vi "Execute.vi"(8 "error in (no error)":errorcluster, 10 "Plugin Display UI in":refnum<class "Plugin Display UI.lvclass">, 11 "Plugin Handler Shifter Data Definition":T1) -> (0 "error out":errorcluster, 1 "Stop?":bool, 2 "Plugin Generic Command out":refnum<class "Plugin Handler Command.lvclass">, 3 "Plugin Handler Shifter Data Out":T1)   [LabVIEW 2011, in "Plugin Display UI.lvclass"]
uses:
  Plugin Display UI.lvclass
  Plugin Handler Command.lvclass
  Plugin Strict Type Definitions/Plugin Handler Shifter Data Definition.ctl
  Parent Plugin Definition/Plugin Template/Generic Plugin.lvclass
  Plugin Strict Type Definitions/Plugin Configuration Information.ctl
  User Interface/UI Command Manager/UI Command Manager.lvclass
  User Interface/UI Command Manager/UI Set Header Text/Set Header Text.lvclass
  User Interface/UI Command Manager/UI Load SubPanel Display/UI Load SubPanel Display.lvclass
  User Interface/UI Command Manager/UI Slide Panel/Slide Panel Off Screen.lvclass
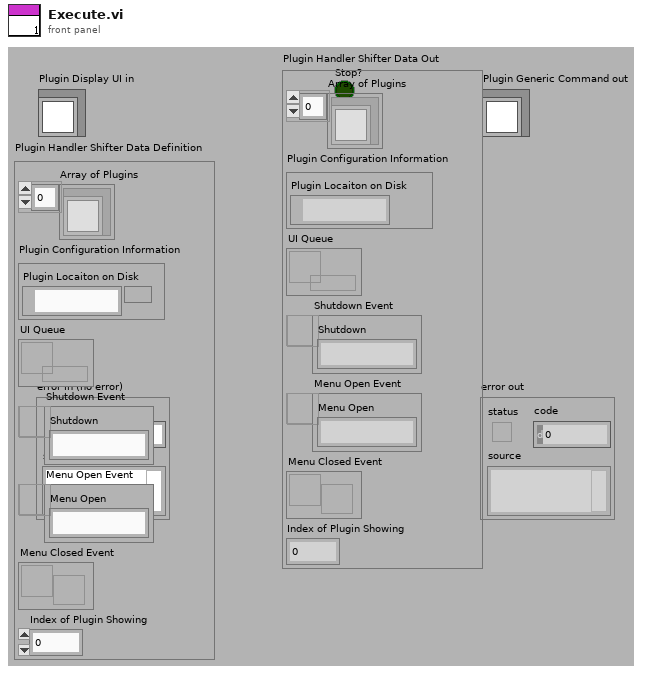
[diagram p1: front panel]
types:
  T1 = typedef "Plugin Handler Shifter Data Definition.ctl" = cluster{"Array of Plugins":refnum<class "Generic Plugin.lvclass">[], "Plugin Configuration Information":T2, "UI Queue":refnum<queue>, "Shutdown Event":refnum<user-event>, "Menu Open Event":refnum<user-event>, "Menu Closed Event":refnum<user-event>, "Index of Plugin Showing":i32}
  T2 = typedef "Plugin Configuration Information.ctl" = cluster{"Plugin Locaiton on Disk":path}
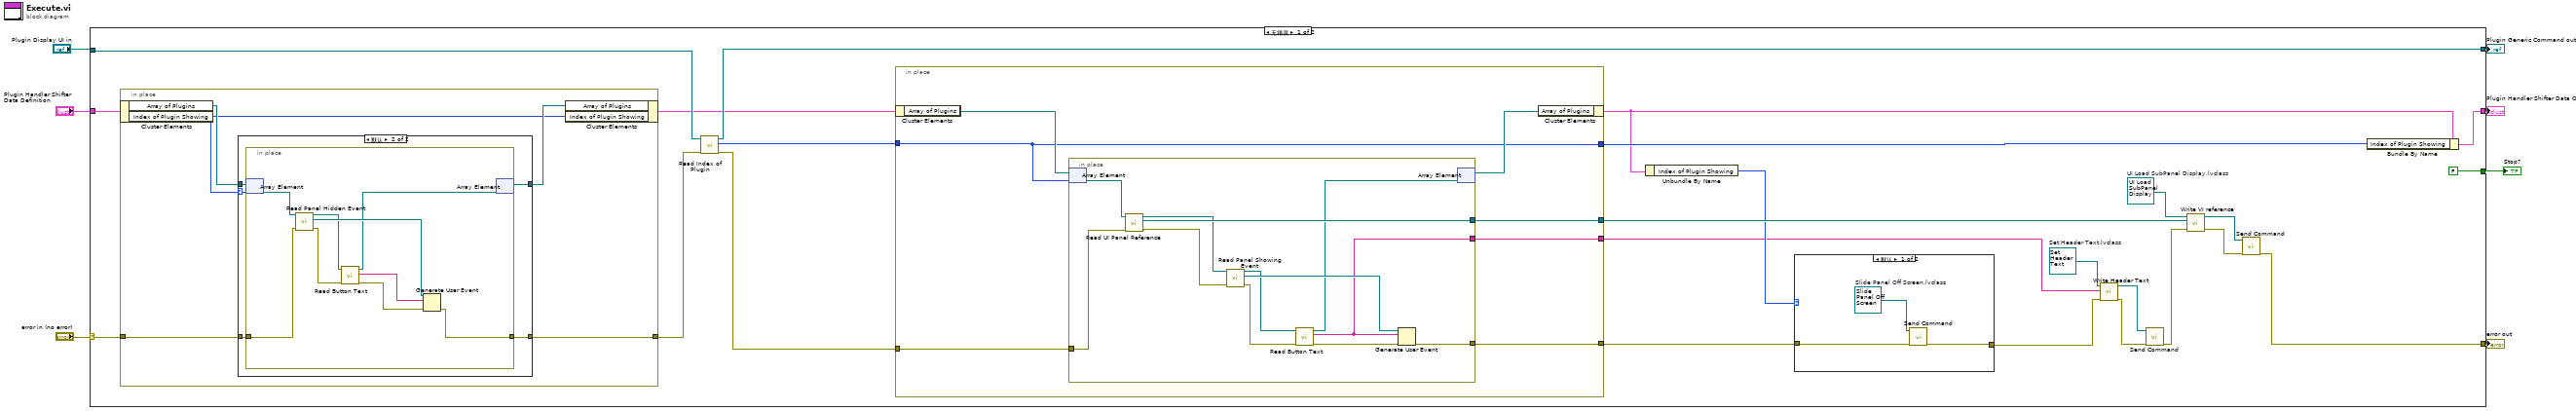
[diagram p0: block diagram]
diagram:
  n1 = case shown="无错误" "error in (no error)" {
    selector: "error in (no error)" -> [w24 w79]
    tunnel: "Plugin Display UI in" -> [w29 w78]
    tunnel: "Plugin Handler Shifter Data Definition" -> [w22 w77]
    tunnel: [w18 w77] -> w6
    tunnel: [w16 w79] -> w2
    tunnel: [w28 w78] -> w3
    tunnel: [FALSE ("Stop?") _] -> w1
    frame No Error {
      w13 = refnum<class "Set Header Text.lvclass"> refnum  # Set Header Text.lvclass
      w32 = refnum<class "UI Load SubPanel Display.lvclass"> refnum  # UI Load SubPanel Display.lvclass
      n2 = in-place {
        in-place-border: w24 -> [w60]
        in-place-border: [w59] -> w23
        n3 = in-place-cluster #1(w22) -> ("Array of Plugins"=w58:refnum<class "Generic Plugin.lvclass">[], "Index of Plugin Showing"=w56:i32)
        n4 = case shown="默认" w56 {
          selector: w56 -> [_ w63]
          tunnel: w60 -> [w61 w67]
          tunnel: [w61 w66] -> w59
          tunnel: w58 -> [w62 w65]
          tunnel: [w62 w64] -> w57
          frame -1 {
          }
          frame Default {
            n5 = in-place {
              in-place-border: w67 -> [w70]
              in-place-border: [w69] -> w66
              n6 = in-place-array #2(w65, w63) -> (w76:refnum<class "Generic Plugin.lvclass">)
              n7 = call "Read Panel Hidden Event.vi"("error in (no error)"=w70, "Generic Plugin in"=w76) -> ("error out"=w71:errorcluster, "Panel Hidden Event"=w74:refnum<user-event>, "Generic Plugin out"=w72:refnum<class "Generic Plugin.lvclass">)  [unwired: 7 in]
              n8 = call-dynamic "Read Button Text.vi"("error in (no error)"=w71, "Generic Plugin in"=w72) -> ("error out"=w73:errorcluster, "Button Text"=w75:string, "Generic Plugin out"=w68:refnum<class "Generic Plugin.lvclass">)  [unwired: 7 in]
              n9 = Generate User Event(user event=w74, event data cluster=w75, error in=w73) -> (error out=w69:errorcluster)  [unwired: 1 out]
              n10 = in-place-array #2(w68) -> (w64:refnum<class "Generic Plugin.lvclass">[])  [unwired: 1 out]
            }
          }
        }
        n11 = in-place-cluster #1("Array of Plugins"=w57, "Index of Plugin Showing"=w56) -> (w21:T1)
      }
      n12 = call "Read Index of Plugin.vi"("error in (no error)"=w23, "Plugin Display UI in"=w29) -> ("error out"=w27:errorcluster, "Index of Plugin"=w20:i32, "Plugin Display UI out"=w28:refnum<class "Plugin Display UI.lvclass">)  [unwired: 7 in]
      n13 = in-place {
        in-place-border: w27 -> [w43]
        in-place-border: [w42] -> w26
        in-place-border: [w41] -> w15
        in-place-border: w20 -> [w38]
        in-place-border: [w38] -> w19
        in-place-border: [w37] -> w11
        n14 = in-place-cluster #3(w21) -> ("Array of Plugins"=w40:refnum<class "Generic Plugin.lvclass">[])
        n15 = in-place {
          in-place-border: w43 -> [w55]
          in-place-border: [w54] -> w42
          in-place-border: [w47] -> w41
          in-place-border: [w44] -> w37
          n16 = in-place-array #4(w40, w38) -> (w46:refnum<class "Generic Plugin.lvclass">)
          n17 = call "Read UI Panel Reference.vi"("error in (no error)"=w55, "Generic Plugin in"=w46) -> ("error out"=w52:errorcluster, "UI Panel Reference"=w54:refnum<vi>, "Generic Plugin out"=w53:refnum<class "Generic Plugin.lvclass">)  [unwired: 7 in]
          n18 = call "Read Panel Showing Event.vi"("error in (no error)"=w52, "Generic Plugin in"=w53) -> ("error out"=w49:errorcluster, "Panel Showing Event"=w51:refnum<user-event>, "Generic Plugin out"=w50:refnum<class "Generic Plugin.lvclass">)  [unwired: 7 in]
          n19 = call-dynamic "Read Button Text.vi"("error in (no error)"=w49, "Generic Plugin in"=w50) -> ("error out"=w48:errorcluster, "Button Text"=w44:string, "Generic Plugin out"=w45:refnum<class "Generic Plugin.lvclass">)  [unwired: 7 in]
          n20 = Generate User Event(user event=w51, event data cluster=w44, error in=w48) -> (error out=w47:errorcluster)  [unwired: 1 out]
          n21 = in-place-array #4(w45) -> (w39:refnum<class "Generic Plugin.lvclass">[])  [unwired: 1 out]
        }
        n22 = in-place-cluster #3("Array of Plugins"=w39) -> (w17:T1)
      }
      n23 = Unbundle By Name(w17) -> ("Index of Plugin Showing"=w14:i32)
      n24 = case shown="默认" w14 {
        tunnel: [w33 w36] -> w9
        tunnel: w15 -> [w34 w36]
        frame Default {
          w35 = refnum<class "Slide Panel Off Screen.lvclass"> refnum  # Slide Panel Off Screen.lvclass
          n25 = call-dynamic "Send Command.vi"("error in (no error)"=w34, "UI Command Manager in"=w35) -> ("error out"=w33:errorcluster)  [unwired: 8 in, 1 out]
        }
        frame -1 {
        }
      }
      n26 = call "Write Header Text.vi"("error in (no error)"=w9, "Header Text"=w11, "Set Header Text in"=w13) -> ("error out"=w10:errorcluster, "Set Header Text out"=w12:refnum<class "Set Header Text.lvclass">)  [unwired: 7 in]
      n27 = call-dynamic "Send Command.vi"("error in (no error)"=w10, "UI Command Manager in"=w12) -> ("error out"=w8:errorcluster)  [unwired: 8 in, 1 out]
      n28 = call-dynamic "Write VI reference.vi"("error in (no error)"=w8, "VI reference"=w26, "UI Load SubPanel Display in"=w32) -> ("error out"=w30:errorcluster, "UI Load SubPanel Display out"=w31:refnum<class "UI Load SubPanel Display.lvclass">)  [unwired: 7 in]
      n29 = call-dynamic "Send Command.vi"("error in (no error)"=w30, "UI Command Manager in"=w31) -> ("error out"=w16:errorcluster)  [unwired: 8 in, 1 out]
      n30 = Bundle By Name(cluster=w17, "Index of Plugin Showing"=w19) -> (w18:T1)
    }
    frame Error {
    }
  }
  "error out" <- w2
  "Plugin Generic Command out" <- w3
  "Stop?" <- w1
  "Plugin Handler Shifter Data Out" <- w6
